vi "Main ActionVIOnLoad.vi"(8 "error in (no error)":errorcluster, 11 "Device Item Ref in":T1 format="%.0x") -> (0 "error out":errorcluster, 3 "Device Item Ref out":T1 format="%.0x")   [LabVIEW 2014, in "SLSC configuration System Explorer.lvlib"]
uses:
  SLSC configuration System Explorer.lvlib
  <vilib>/NI Veristand/Custom Device API/Custom Device Item Ref.ctl
  NationalInstruments.VeriStand.SystemDefinitionAPI
  Shared/Constants.vi
  <vilib>/NI Veristand/Custom Device API/Custom Device API.lvlib
  Shared/SLSC configuration Shared.lvlib
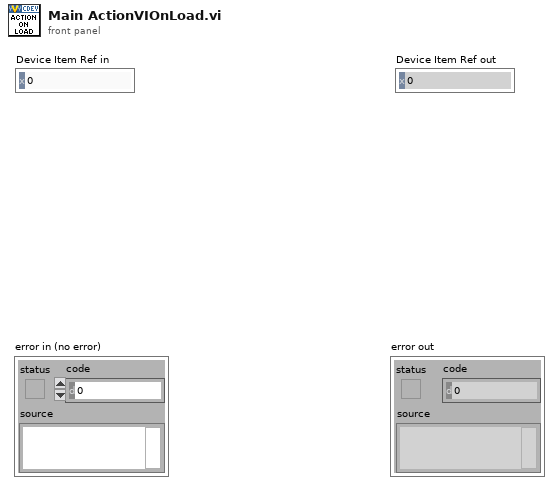
[diagram p1: front panel]
types:
  T1 = typedef "Custom Device API.lvlib/Custom Device Item Ref.ctl" = u64
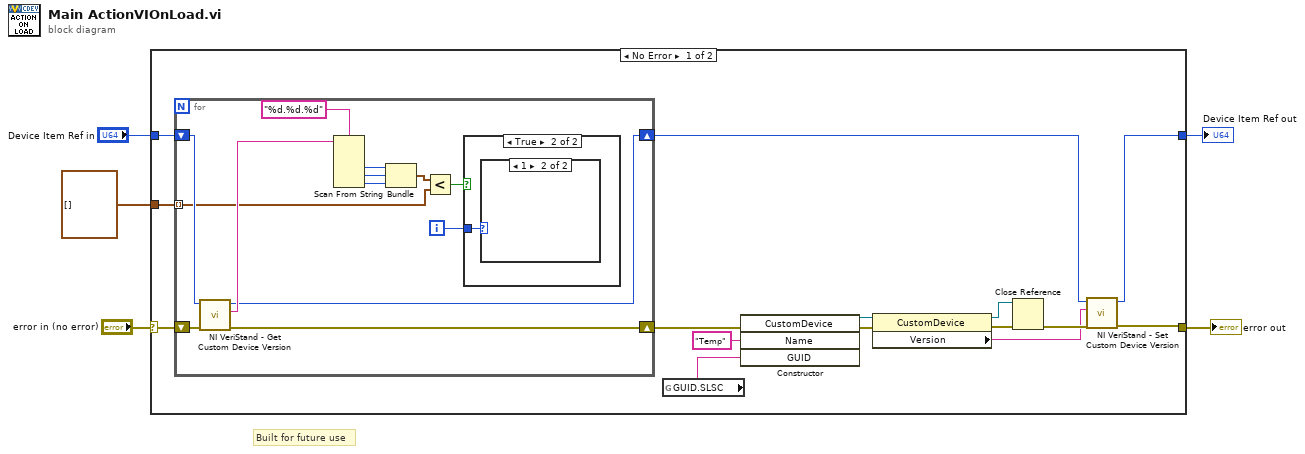
[diagram p0: block diagram]
diagram:
  # "Built for future use"
  n1 = case shown="No Error" "error in (no error)" {
    selector: "error in (no error)" -> [w18 w36]
    tunnel: [w7 w36] -> w2
    tunnel: "Device Item Ref in" -> [w19 w35]
    tunnel: cluster{"Major":i32, "Minor":i32, "Fix":i32}[] [] -> [w20 _]
    tunnel: [w6 w35] -> w1
    frame No Error {
      n2 = for {
        tunnel: w20 -> [w25] mode=indexing
        shift-right: [w22] -> w9
        shift-left: w19 -> [w32]
        shift-right: [w21] -> w17
        shift-left: w18 -> [w33]
        i -> [w23]
        n3 = call <vilib>:"NI VeriStand - Get Custom Device Version.vi"("error in (no error)"=w33, "Device Ref in"=w32) -> ("error out"=w21:errorcluster, "Value"=w30:string, "Device Ref out"=w22:T1)  [unwired: 7 in]
        n4 = Scan From String(format string="%d.%d.%d", input string=w30) -> (output 1=w29:i32, output 2=w28:i32, output 3=w27:i32)  [unwired: 5 in, 3 out]
        n5 = Bundle(w29, w28, w27) -> (w26:cluster{i32, i32, i32})  [unwired: 1 in]
        n6 = Less?(x=w26, y=w25) -> (x < y?=w24:bool)
        n7 = case shown="True" w24 {
          tunnel: w23 -> [_ w34]
          frame False {
          }
          frame True {
            n8 = case shown="1" w34 {
              frame 0, Default {
              }
              frame 1 {
              }
            }
          }
        }
      }
      n9 = global read "Constants.vi" "GUID.SLSC"() -> (w15:string)
      n10 = constructor class="CustomDevice"(error in=w17, "Name"="Temp", "GUID"=w15) -> (reference out=w13:refnum<k24>, error out=w14:errorcluster)  [unwired: 2 in, 3 out]
      n11 = property class="CustomDevice"(reference=w13, error in=w14) -> (reference out=w11:refnum<k24>, error out=w12:errorcluster, "Version"=w8:string)
      n12 = Close Reference(reference=w11, error in (no error)=w12) -> (error out=w10:errorcluster)
      n13 = call <vilib>:"NI VeriStand - Set Custom Device Version.vi"("error in (no error)"=w10, "Value"=w8, "Device Ref in"=w9) -> ("error out"=w7:errorcluster, "Device Ref out"=w6:T1)  [unwired: 7 in]
    }
    frame Error {
    }
  }
  "error out" <- w2
  "Device Item Ref out" <- w1
